vi "setREF_phi.vi"(8 "error in (no error)":errorcluster, 9 "Phase (°)":dbl, 10 "REF Channel":i32=1 min=1 max=16, 11 "Instrument.LockinAPI in":refnum<class "Instrument.LockinAPI.lvclass">) -> (0 "error out":errorcluster, 3 "Instrument.LockinAPI out":refnum<class "Instrument.LockinAPI.lvclass">)   [LabVIEW 2019, in "Instrument.LockinAPI.lvclass"]
doc: "API to configure a REF phase.\n\nSpecify which channel you want to change and the value you want to set.\n\nIf address=\"\", this API reads from localhost\nIf address is remote lockin, you need to add this computer to allowed whitelist on the lockin computer you are trying to access."
uses:
  Instrument.LockinAPI.lvclass
  C:/Users/patrick/Documents/GitHub/Instrument-Framework/lvsrc/Framework/Instrument/Instrument.lvclass
  Typedefs/LockinAPI.commands--Enum.ctl
  Typedefs/LockinAPI.REF_phi--cluster.ctl
  Instrument/Instrument.lvclass
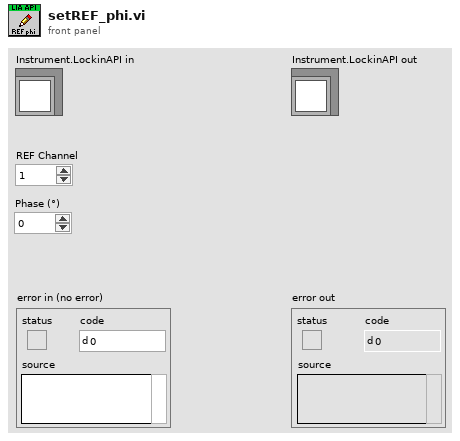
[diagram p1: front panel]
types:
  T1 = typedef "Instrument.LockinAPI.lvclass/LockinAPI.REF_phi--cluster.ctl" = cluster{"REF Channel":i32, "Phase (°)":dbl}
  T2 = typedef "Instrument.LockinAPI.lvclass/LockinAPI.commands--Enum.ctl" = enum16{"setAI", "setAO", "setAO_Amplitude", "setAO_DC", "setAO_Frequency", "setAO_Phase", "setAO_Function", "setAO_I+", "setREF", "setREF_Frequency", "setREF_Phase", "setREF_TC", "setREF_Roll-Off", "setDAQ", "setSampling", "setOffset", "setState", "getState", "getAO", "getAI", "getResults", "getSampling", "getAOconfig", "getREFconfig", "setInputGain", "setOutputGain", "getInputGain", "getOutputGain", "setSamplingMode", "getSamplingMode", "setSweep", "setSweepTime", "setSweepTable", "getStatus", "getSweepResults", "getSweepWaveforms", "startSweep", "stopSweep", "setAUX", "getAUX"}
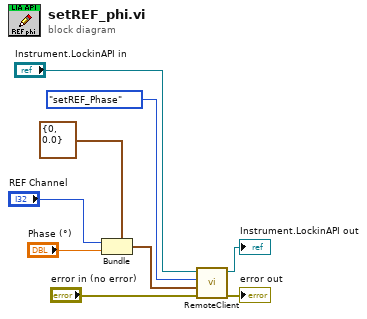
[diagram p0: block diagram]
diagram:
  n1 = Bundle(cluster=T1 {"REF Channel"=0, "Phase (°)"=0.0} ("setREF_phi"), "REF Channel"="REF Channel", "Phase (°)"="Phase (°)") -> (w9:T1)
  n2 = call "RemoteClient.vi"("error in (no error)"="error in (no error)", "Data in"=w9, "Command in"=LockinAPI.commands--Enum."setREF_Phase" ("Command"), "Instrument in"="Instrument.LockinAPI in") -> ("error out"=→"error out":errorcluster, "Instrument out"=→"Instrument.LockinAPI out":refnum<class "Instrument.LockinAPI.lvclass">)  [unwired: 4 in, 2 out]
